vi "ScriptCommands.vi"(11 "Auton Routines":T1[](array[typedef])) -> ()   [LabVIEW 2013]
uses:
  Command Type.ctl
  <vilib>/Rock Robotics/WPI/RobotDrive/WPI_RobotDriveGetSetRefNum.vi
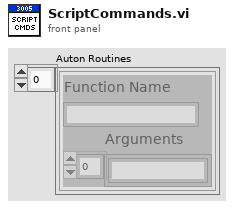
[diagram p1: front panel]
types:
  T1 = typedef "Command Type.ctl" = cluster{"Function Name":string, "Arguments":string[]}
  T2 = typedef "WPI_EncoderDevRef.ctl" = cluster{"DevStatus":errorcluster, "EncoderIndex":T3, "CounterIndex":T4, "DistancePerCount":dbl, "Decoding Type":T5}
  T3 = typedef "FPGA_EncoderIdx.ctl" = enum8{"Enc 0", "Enc 1", "Enc 2", "Enc 3", "Invalid"}
  T4 = typedef "FPGA_CounterCtrSystemIndex.ctl" = enum8{"Ctr 0", "Ctr 1", "Ctr 2", "Ctr 3", "Ctr 4", "Ctr 5", "Ctr 6", "Ctr 7", "Invalid"}
  T5 = typedef "WPI_EncoderType.ctl" = enum16{"1x", "2x", "4x"}
  T6 = typedef "WPI_RobotDriveDevRef.ctl" = cluster{"DevStatus":errorcluster, "Motors[]":T7[], "Square Inputs":bool, "Max Output":dbl, "Isochronous":bool}
  T7 = typedef "WPI_MotorControlDeviceRef.ctl" = cluster{"DeviceStatus":errorcluster, "Type":enum16{"PWM", "CAN"}, "PWM":cluster{"Digital Module":T8, "PWM Channel":T9, "DeadBand":T10}, "CAN":cluster{"Device Number":u8, "Control Mode":T11, "Semaphore":T12, "Max Vout":dbl}, "Invert":bool, "TransformRef":T13, "InvTransformRef":T13}
  T8 = typedef "FPGA_TypedefDigitalModule.ctl" = enum16{"Digital Module 1", "Digital Module 2"}
  T9 = typedef "FPGA_DIOPWMChannel.ctl" = enum8{"PWM 1", "PWM 2", "PWM 3", "PWM 4", "PWM 5", "PWM 6", "PWM 7", "PWM 8", "PWM 9", "PWM 10", "Invalid"}
  T10 = typedef "WPI_PWMDeadband.ctl" = cluster{"Name":string, "maxPositivePwm":i32, "minPositivePwm":i32, "centerPwm":i32, "maxNegativePwm":i32, "minNegativePwm":i32, "angularRange":u16}
  T11 = typedef "WPI_CANJaguar_ControlMode.ctl" = enum8{"Percent VBus", "Current", "Speed", "Position", "Voltage"}
  T12 = typedef "Semaphore RefNum" = refnum<k1>
  T13 = typedef "WPI_PWMTransform_ConPane.ctl" = refnum<vi>
  T14 = typedef "WPI_CounterDevRef.ctl" = cluster{"DevStatus":errorcluster, "CntIndex":T4}
  T15 = typedef "WPI_GyroDevRef.ctl" = cluster{"DevStatus":errorcluster, "Analog Module":T16, "Analog Channel":T17, "Offset":dbl, "Gain (VoltsPerDegree/Second)":dbl}
  T16 = typedef "FPGA_TypedefAnalogModule.ctl" = enum16{"Analog Module 1", "Analog Module 2"}
  T17 = typedef "FPGA_AIChannel.ctl" = enum8{"AI 1", "AI 2", "AI 3", "AI 4", "AI 5", "AI 6", "AI 7", "AI 8", "Invalid"}
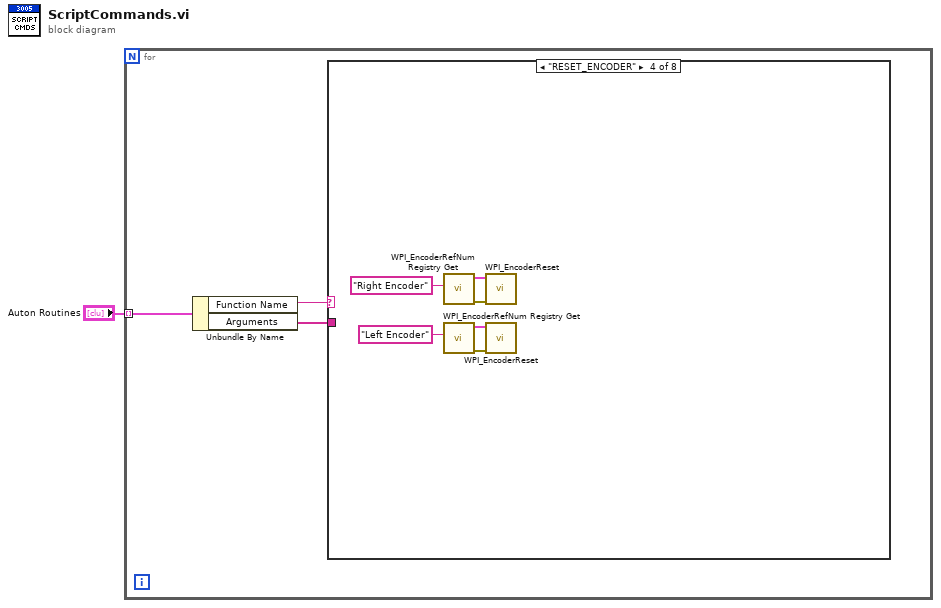
[diagram p0: block diagram]
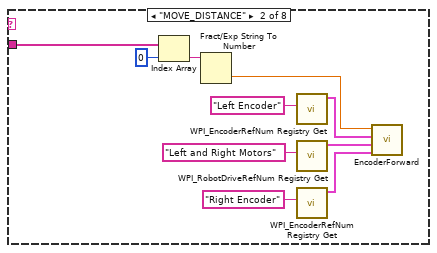
[diagram p3: hidden frame]
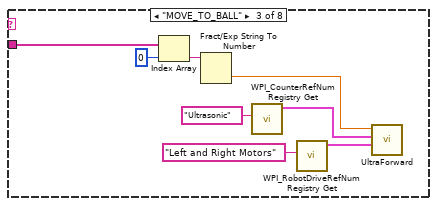
[diagram p4: hidden frame]
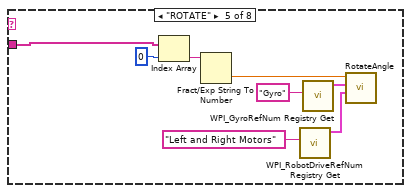
[diagram p5: hidden frame]
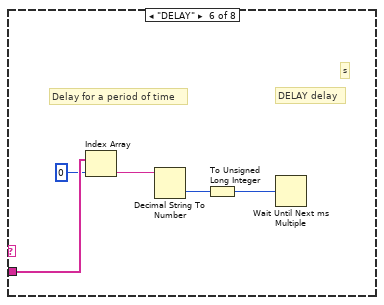
[diagram p6: hidden frame]
diagram:
  n1 = for {
    tunnel: "Auton Routines" -> [w4] mode=indexing
    n2 = Unbundle By Name(w4) -> ("Function Name"=w3:string, "Arguments"=w2:string[])
    n3 = case shown="\"RESET_ENCODER\"" w3 {
      tunnel: w2 -> [_ w14 w22 _ w36 w41 _ _]
      frame Default {
      }
      frame "MOVE_DISTANCE" {
        n4 = Index Array(array=w14, index=0) -> (element=w12:string)
        n5 = Fract/Exp String To Number(string=w12) -> (number=w5:dbl)  [unwired: 3 in, 1 out]
        n6 = call <vilib>:"WPI_EncoderRefNum Registry Get.vi"("refnum name"="Left Encoder") -> ("EncoderDevRef"=w6:T2)  [unwired: 9 in, 1 out]
        n7 = call <vilib>:"WPI_RobotDriveRefNum Registry Get.vi"("refnum name"="Left and Right Motors") -> ("RobotDriveDevRef"=w10:T6)  [unwired: 1 in, 9 out]
        n8 = call <vilib>:"WPI_EncoderRefNum Registry Get.vi"("refnum name"="Right Encoder") -> ("EncoderDevRef"=w7:T2)  [unwired: 9 in, 1 out]
        n9 = call "EncoderForward.vi"("EncoderDevRef 4"=w7, "RobotDriveDevRef"=w10, "EncoderDevRef"=w6, "Target"=w5) -> ()  [unwired: 5 in, 3 out]
      }
      frame "MOVE_TO_BALL" {
        n10 = Index Array(array=w22, index=0) -> (element=w20:string)
        n11 = Fract/Exp String To Number(string=w20) -> (number=w17:dbl)  [unwired: 3 in, 1 out]
        n12 = call <vilib>:"WPI_CounterRefNum Registry Get.vi"("refnum name"="Ultrasonic") -> ("CounterDevRef"=w16:T14)  [unwired: 9 in, 1 out]
        n13 = call <vilib>:"WPI_RobotDriveRefNum Registry Get.vi"("refnum name"="Left and Right Motors") -> ("RobotDriveDevRef"=w18:T6)  [unwired: 1 in, 9 out]
        n14 = call "UltraForward.vi"("RobotDriveDevRef"=w18, "CounterDevRef in"=w16, "Target"=w17) -> ()  [unwired: 8 in, 1 out]
      }
      frame "RESET_ENCODER" {
        n15 = call <vilib>:"WPI_EncoderRefNum Registry Get.vi"("refnum name"="Right Encoder") -> ("error out"=w28:errorcluster, "EncoderDevRef"=w27:T2)  [unwired: 9 in]
        n16 = call <vilib>:"WPI_EncoderRefNum Registry Get.vi"("refnum name"="Left Encoder") -> ("error out"=w23:errorcluster, "EncoderDevRef"=w24:T2)  [unwired: 9 in]
        n17 = call <vilib>:"WPI_EncoderReset.vi"("error in (no error)"=w28, "EncoderDevRef"=w27) -> ()  [unwired: 8 in, 2 out]
        n18 = call <vilib>:"WPI_EncoderReset.vi"("error in (no error)"=w23, "EncoderDevRef"=w24) -> ()  [unwired: 8 in, 2 out]
      }
      frame "ROTATE" {
        n19 = Index Array(array=w36, index=0) -> (element=w34:string)
        n20 = Fract/Exp String To Number(string=w34) -> (number=w29:dbl)  [unwired: 3 in, 1 out]
        n21 = call <vilib>:"WPI_RobotDriveRefNum Registry Get.vi"("refnum name"="Left and Right Motors") -> ("RobotDriveDevRef"=w30:T6)  [unwired: 1 in, 9 out]
        n22 = call <vilib>:"WPI_GyroRefNum Registry Get.vi"("refnum name"="Gyro") -> ("GyroDevRef"=w33:T15)  [unwired: 9 in, 1 out]
        n23 = call "RotateAngle.vi"("RobotDriveDevRef"=w30, "GyroDevRef"=w33, "Target"=w29) -> ()  [unwired: 7 in, 2 out]
      }
      frame "DELAY" {
        # "Delay for a period of time"
        # "s"
        # "DELAY delay"
        n24 = Index Array(array=w41, index=0) -> (element=w39:string)
        n25 = Decimal String To Number(string=w39) -> (number=w38:i32)  [unwired: 2 in, 1 out]
        n26 = To Unsigned Long Integer(number=w38) -> (unsigned 32bit integer=w37:u32)
        n27 = Wait Until Next ms Multiple(millisecond multiple=w37) -> ()  [unwired: 1 out]
      }
      frame "DETECT_HOT_GOAL" {
      }
      frame "STOP" {
      }
    }
  }
